vi "Correct_RD_Files.vi"() -> ()   [LabVIEW 2010]
panel:
  out "error out":errorcluster
  out "Number of strings found":i32
  out "Current File Number":i32
  out "No of Files Changed":i32
  out "Current FIlename":path
  in  "stop":bool
  out "Total Number of Files":i32
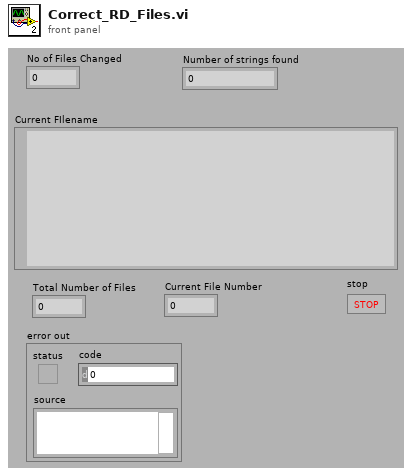
[diagram p1: front panel]
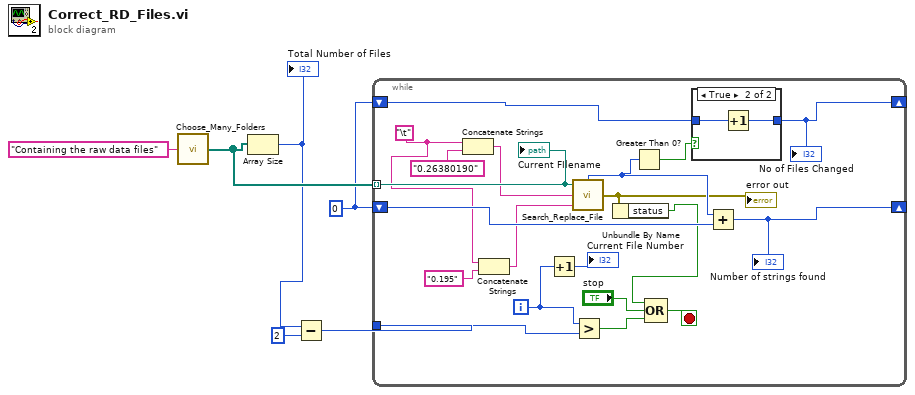
[diagram p0: block diagram]
diagram:
  w2 = 0
  n1 = call "Choose_Many_Folders.vi"("Purpose of choosing folder"="Containing the raw data files") -> ("Files"=w6:path[])
  n2 = Array Size(array=w6) -> (size(s)=w4:i32)
  "Total Number of Files" <- w4
  n3 = Subtract(x=w4, y=2) -> (x-y=w5:i32)
  n4 = while {
    tunnel: w6 -> [w26] mode=indexing
    tunnel: w5 -> [w25]
    shift-right: [w21] -> _
    shift-left: w2 -> [w20]
    shift-right: [w16] -> _
    shift-left: w2 -> [w17]
    i -> [w15]
    stop <- w22 stop-if-true
    w9 = "\t"
    n5 = Concatenate Strings(w9, "0.26380190" ("Search_String")) -> (w10:string)
    n6 = Concatenate Strings(w9, "0.195" ("Replace_String")) -> (w7:string)
    n7 = Increment(x=w15) -> (x+1=→"Current File Number":i32)
    n8 = call "Search_Replace_File.vi"("Replace_String"=w7, "Search_String"=w10, "Path"=w26) -> ("error out"=w13:errorcluster, "Number Found"=w19:i32)
    "error out" <- w13
    n9 = Greater?(x=w15, y=w25) -> (0:w24:bool)
    n10 = Unbundle By Name(w13) -> ("status"=w12:bool)
    n11 = Greater Than 0?(x=w19) -> (x > 0?=w18:bool)
    n12 = Compound Arithmetic op=OR(w12, "stop", w24) -> (w22:bool)
    n13 = case shown="True" w18 {
      tunnel: w17 -> [w27 w29]
      tunnel: [w27 w28] -> w16
      frame False {
      }
      frame True {
        n14 = Increment(x=w29) -> (x+1=w28:i32)
      }
    }
    "No of Files Changed" <- w16
    n15 = Add(x=w19, y=w20) -> (x+y=w21:i32)
    "Number of strings found" <- w21
    "Current FIlename" <- w26
  }
